vi "F_compareBMS_B.vi"(6 "错误输入（无错误）":errorcluster, 8 "pa_BMS_ID_S":string, 9 "引用输入":refnum<k24>) -> (0 "错误输出":errorcluster, 2 "F_CompareBMS_B":bool, 3 "引用输出":refnum<k24>)   [LabVIEW 2013]
uses:
  AuthorizationToolClassLibrary.dll
panel:
  # "对比BMS编号"
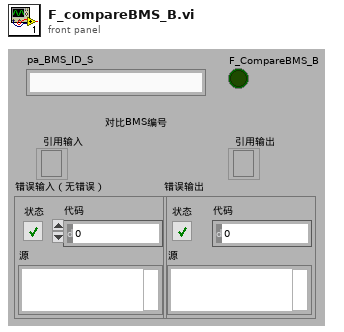
[diagram p1: front panel]
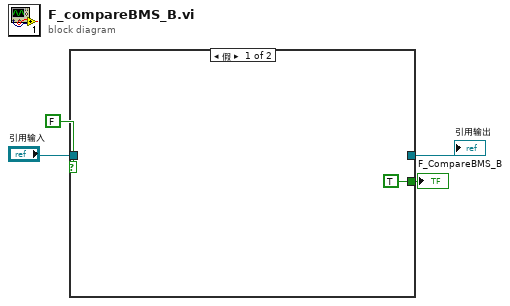
[diagram p0: block diagram]
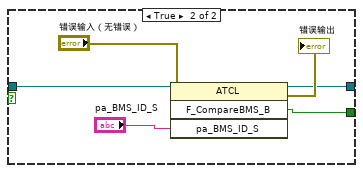
[diagram p2: hidden frame]
diagram:
  n1 = case shown="假" FALSE {
    tunnel: [TRUE ("F_CompareBMS_B") w11] -> w4
    tunnel: [_ w7] -> w3
    tunnel: "引用输入" -> [_ w6]
    frame False {
    }
    frame True {
      n2 = invoke class="ATCL" method="F_CompareBMS_B"(reference=w6, error in="错误输入（无错误）", "pa_BMS_ID_S"="pa_BMS_ID_S") -> (reference out=w7:refnum<k24>, error out=→"错误输出":errorcluster, "F_CompareBMS_B"=w11:bool)  [unwired: 1 in, 1 out]
    }
  }
  "F_CompareBMS_B" <- w4
  "引用输出" <- w3
